vi "Trim Whitespace (String)__ogtk.vi"(5 "remove (leading and trailing)":enum16{"leading", "trailing", "both"}(ring)=enum."both", 6 "String in":string) -> (1 "String out":string)   [LabVIEW 2011]
doc: "Removes leading and/or trailing whitespace from a string. Whitespace is defined as any of the following \\t \\n \\0B \\f \\r"
panel:
  # "[OpenG VI Tags] ***Do Not Remove***"
  # "Trim Whitespace.vi\n\nRemoves leading and/or trailing whitespace from a string.\n\nPlease visit http://www.OpenG.org to learn about the\nOpen Source LabVIEW software movement.\n\nNOTICE -- YOU MUST LEAVE THIS NOTICE IN PLACE.  PER THE TERMS OF THE LICENSE BELOW, YOU MAY SUBLICENSE THIS SOFTWARE \nIN ANY WAY THAT DOES NOT CONFLICT WITH THIS LICENSE.\n\n### BSD License (http://www.opensource.org/licenses/bsd-license.php) Begin ###\n \nCopyright (c) 2002-2006, Jim Kring <jim@jimkring.com>\nCopyright (c) 2002, Cal-Bay Systems, Inc. <info@calbay.com>\n\nAll rights reserved.\n\nRedistribution and use in source and binary forms, with or without modification, are permitted provided that the following conditions are met:\n\n    * Redistributions of source code must retain the above copyright notice, this list of conditions and the following disclaimer.\n    * Redistributions in binary form must reproduce the above copyright notice, this list of conditions and the following disclaimer in the \n       documentation and/or other materials provided with the distribution.\n    * Neither the name of SciWare, James Kring, Inc., nor the names of its contributors may be used to endorse or promote products derived \n       from this software without specific prior written permission.\n\nTHIS SOFTWARE IS PROVIDED BY THE COPYRIGHT HOLDERS AND CONTRIBUTORS \"AS IS\" AND ANY EXPRESS OR IMPLIED WARRANTIES, \nINCLUDING, BUT NOT LIMITED TO, THE IMPLIED WARRANTIES OF MERCHANTABILITY AND FITNESS FOR A PARTICULAR PURPOSE ARE \nDISCLAIMED. IN NO EVENT SHALL THE COPYRIGHT OWNER OR CONTRIBUTORS BE LIABLE FOR ANY DIRECT, INDIRECT, INCIDENTAL,\n SPECIAL, EXEMPLARY, OR CONSEQUENTIAL DAMAGES (INCLUDING, BUT NOT LIMITED TO, PROCUREMENT OF SUBSTITUTE GOODS OR \nSERVICES; LOSS OF USE, DATA, OR PROFITS; OR BUSINESS INTERRUPTION) HOWEVER CAUSED AND ON ANY THEORY OF LIABILITY, \nWHETHER IN CONTRACT, STRICT LIABILITY, OR TORT (INCLUDING NEGLIGENCE OR OTHERWISE) ARISING IN ANY WAY OUT OF THE USE \nOF THIS SOFTWARE, EVEN IF ADVISED OF THE POSSIBILITY OF SUCH DAMAGE.\n\n### BSD License End ###"
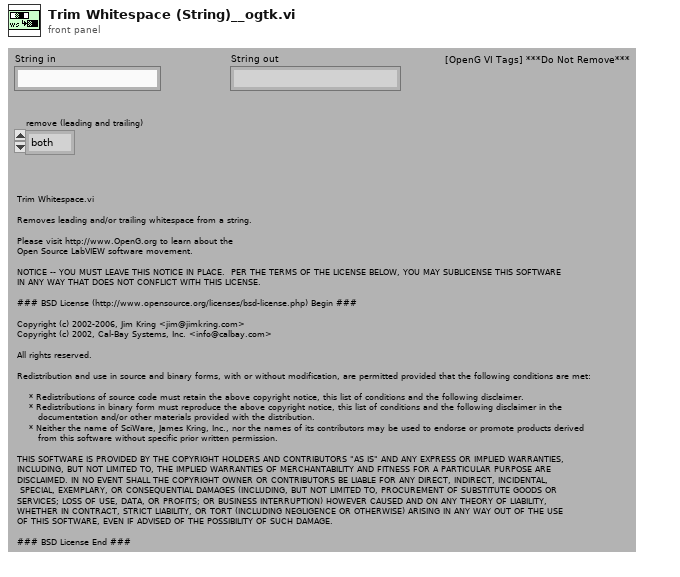
[diagram p1: front panel]
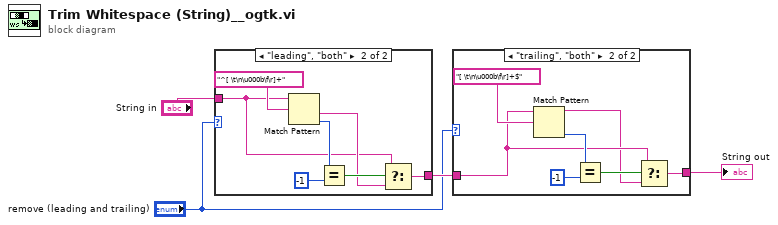
[diagram p0: block diagram]
diagram:
  n1 = case shown="\"leading\", \"both\"" "remove (leading and trailing)" {
    tunnel: [w5 w7] -> w4
    tunnel: "String in" -> [w5 w6]
    frame "trailing" {
    }
    frame "leading", "both" {
      n2 = Match Pattern(string=w6, regular expression="^[ \t\n\u000b\f\r]+") -> (after substring=w8:string, offset past match=w11:i32)  [unwired: 1 in, 2 out]
      n3 = Equal?(x=w11, y=-1) -> (x = y?=w9:bool)
      n4 = Select(t=w6, s=w9, f=w8) -> (s? t:f=w7:string)
    }
  }
  n5 = case shown="\"trailing\", \"both\"" "remove (leading and trailing)" {
    tunnel: w4 -> [w13 w16]
    tunnel: [w13 w14] -> w3
    frame "leading" {
    }
    frame "trailing", "both" {
      n6 = Match Pattern(string=w16, regular expression="[ \t\n\u000b\f\r]+$") -> (before substring=w15:string, offset past match=w17:i32)  [unwired: 1 in, 2 out]
      n7 = Equal?(x=w17, y=-1) -> (x = y?=w19:bool)
      n8 = Select(t=w16, s=w19, f=w15) -> (s? t:f=w14:string)
    }
  }
  "String out" <- w3
